vi "LSX Set TVR Out Resolution.vi"(6 "lR":i32, 7 "lZ":i32, 8 "error in (no error)":errorcluster, 9 "lY":i32, 10 "lX":i32, 11 "lLSID":i32) -> (0 "error out":errorcluster, 3 "function return":i32)   [LabVIEW 2018, in "Tango.lvlib"]
doc: "TANGOAPI int TANGOCALL LSX_SetTVROutResolution (int lLSID, int lX, int lY, int lZ, int lR);"
uses:
  <userlib>/Tango/Tango.lvlib
  <userlib>/Tango/Tango_DLL.dll
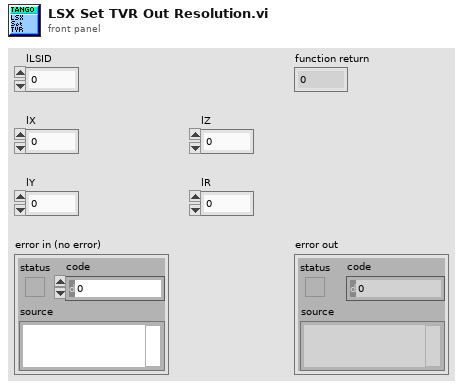
[diagram p1: front panel]
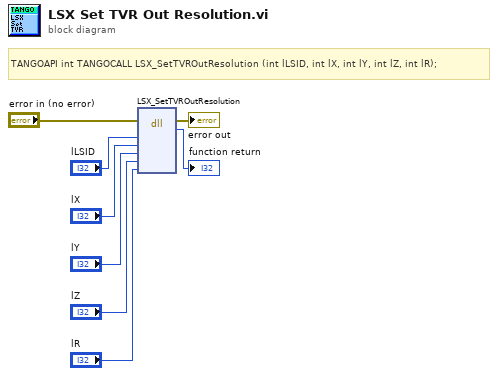
[diagram p0: block diagram]
diagram:
  # "TANGOAPI int TANGOCALL LSX_SetTVROutResolution (int lLSID, int lX, int lY, int lZ, int lR);"
  n1 = dll-call lib="C:/Program Files (x86)/National Instruments/LabVIEW 2018/user.lib/Tango/Tango_DLL.*" fn="LSX_SetTVROutResolution"(error in="error in (no error)", "lLSID"="lLSID", "lX"="lX", "lY"="lY", "lZ"="lZ", "lR"="lR") -> (error out=→"error out":errorcluster, →"function return":i32)  [unwired: 7 in, 1 out]
